vi "TH_Ini_ReadParameters.vi"() -> (19 "error out":errorcluster)   [LabVIEW 2020]
uses:
  TH_StartParameters.vi
  <vilib>/Utility/config.llb/Read Key (String).vi
  TH_Ini_Parameters.vi
  <vilib>/Utility/config.llb/Read Key (Boolean).vi
  <vilib>/Utility/config.llb/Read Key (I32).vi
  <vilib>/Utility/config.llb/NI_LVConfig.lvlib
panel:
  out "Inifile Path":path
  out "Vi Path":path
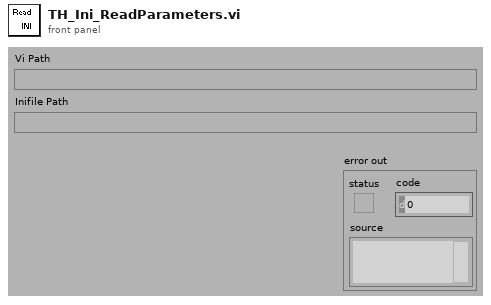
[diagram p1: front panel]
types:
  T1 = typedef "NI_LVConfig.lvlib/Config Data RefNum.ctl" = refnum<k1>
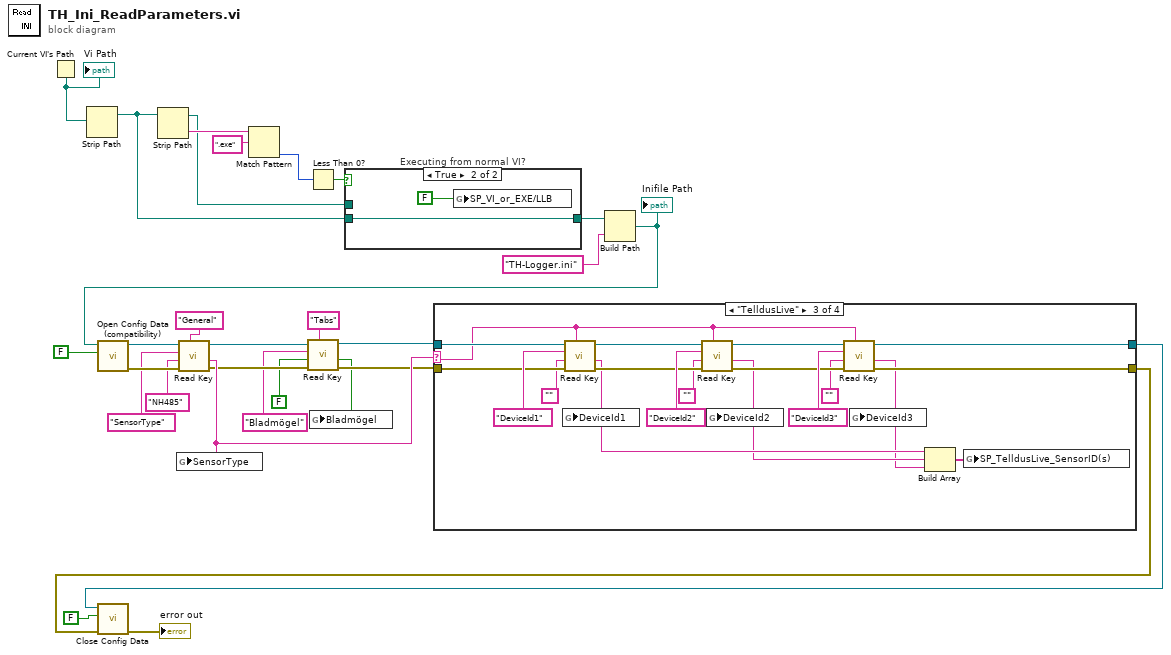
[diagram p0: block diagram]
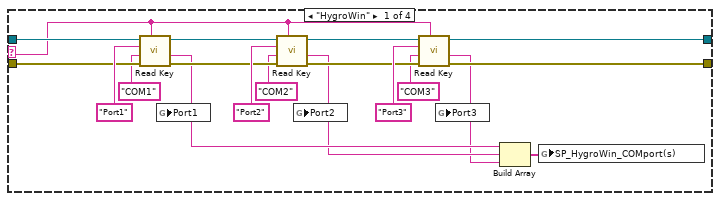
[diagram p2: hidden frame]
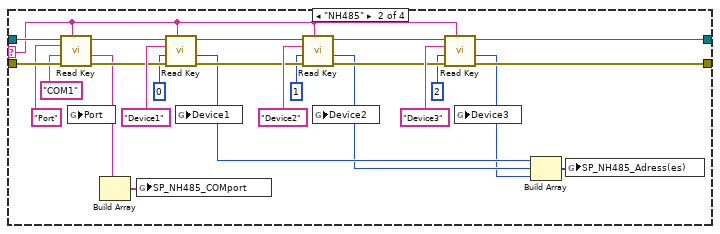
[diagram p3: hidden frame]
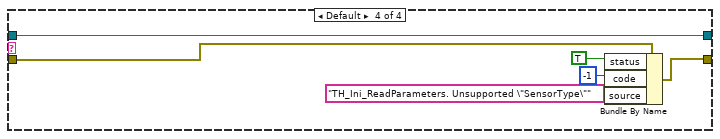
[diagram p4: hidden frame]
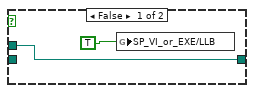
[diagram p5: hidden frame]
diagram:
  n1 = Current VI's Path() -> (path=w27:path)
  "Vi Path" <- w27
  n2 = Strip Path(path=w27) -> (stripped path=w24:path)  [unwired: 1 out]
  n3 = Strip Path(path=w24) -> (stripped path=w23:path, name=w29:string)
  n4 = Match Pattern(string=w29, regular expression=".exe") -> (offset past match=w25:i32)  [unwired: 1 in, 3 out]
  n5 = Less Than 0?(x=w25) -> (x < 0?=w26:bool)
  n6 = case "Executing from normal VI?" shown="True" w26 {
    tunnel: w24 -> [_ w33]
    tunnel: w23 -> [w31 _]
    tunnel: [w31 w33] -> w22
    frame False {
      n7 = global write "TH_StartParameters.vi" "SP_VI_or_EXE/LLB"(TRUE) -> ()
    }
    frame True {
      n8 = global write "TH_StartParameters.vi" "SP_VI_or_EXE/LLB"(FALSE) -> ()
    }
  }
  n9 = Build Path(base path=w22, name or relative path="TH-Logger.ini") -> (appended path=w18:path)
  "Inifile Path" <- w18
  n10 = call <vilib>:"Open Config Data (compatibility).vi"("create file if necessary (T)"=FALSE ("create file if necessary? (T)"), "configuration file path"=w18) -> ("error out"=w17:errorcluster, "refnum"=w16:T1)  [unwired: 7 in, 1 out]
  n11 = call-poly <vilib>:"Read Key.vi"("section"="General", "error in (no error)"=w17, "default value"="NH485", "key"="SensorType", "refnum"=w16) -> ("error out"=w7:errorcluster, "value"=w14:string, "refnum out"=w10:T1)  [unwired: 3 in, 1 out]
  n12 = global write "TH_Ini_Parameters.vi" "SensorType"(w14) -> ()
  n13 = call-poly <vilib>:"Read Key.vi"("section"="Tabs", "error in (no error)"=w7, "default value"=FALSE, "key"="Bladmögel", "refnum"=w10) -> ("error out"=w8:errorcluster, "value"=w4:bool, "refnum out"=w9:T1)  [unwired: 3 in, 1 out]
  n14 = global write "TH_Ini_Parameters.vi" "Bladmögel"(w4) -> ()
  n15 = case shown="\"TelldusLive\"" w14 {
    selector: w14 -> [w43 w63 w87 _]
    tunnel: w9 -> [w45 w77 w89 w102]
    tunnel: w8 -> [w44 w76 w88 w100]
    tunnel: [w42 w65 w86 w102] -> w12
    tunnel: [w41 w64 w85 w101] -> w13
    frame "HygroWin" {
      n16 = call-poly <vilib>:"Read Key.vi"("section"=w43, "error in (no error)"=w44, "default value"="COM1", "key"="Port1", "refnum"=w45) -> ("error out"=w49:errorcluster, "value"=w40:string, "refnum out"=w50:T1)  [unwired: 3 in, 1 out]
      n17 = global write "TH_Ini_Parameters.vi" "Port1"(w40) -> ()
      n18 = call-poly <vilib>:"Read Key.vi"("section"=w43, "error in (no error)"=w49, "default value"="COM2", "key"="Port2", "refnum"=w50) -> ("error out"=w46:errorcluster, "value"=w39:string, "refnum out"=w47:T1)  [unwired: 3 in, 1 out]
      n19 = global write "TH_Ini_Parameters.vi" "Port2"(w39) -> ()
      n20 = call-poly <vilib>:"Read Key.vi"("section"=w43, "error in (no error)"=w46, "default value"="COM3", "key"="Port3", "refnum"=w47) -> ("error out"=w41:errorcluster, "value"=w38:string, "refnum out"=w42:T1)  [unwired: 3 in, 1 out]
      n21 = global write "TH_Ini_Parameters.vi" "Port3"(w38) -> ()
      n22 = Build Array(w40, w39, w38) -> (w37:string[])
      n23 = global write "TH_StartParameters.vi" "SP_HygroWin_COMport(s)"(w37) -> ()
    }
    frame "NH485" {
      n24 = call-poly <vilib>:"Read Key.vi"("section"=w63, "error in (no error)"=w76, "default value"="COM1", "key"="Port", "refnum"=w77) -> ("error out"=w72:errorcluster, "value"=w62:string, "refnum out"=w73:T1)  [unwired: 3 in, 1 out]
      n25 = global write "TH_Ini_Parameters.vi" "Port"(w62) -> ()
      n26 = Build Array(w62, w62, w62) -> (w61:string[])
      n27 = global write "TH_StartParameters.vi" "SP_NH485_COMport"(w61) -> ()
      n28 = call-poly <vilib>:"Read Key.vi"("section"=w63, "error in (no error)"=w72, "default value"=0, "key"="Device1", "refnum"=w73) -> ("error out"=w69:errorcluster, "value"=w60:i32, "refnum out"=w70:T1)  [unwired: 3 in, 1 out]
      n29 = global write "TH_Ini_Parameters.vi" "Device1"(w60) -> ()
      n30 = call-poly <vilib>:"Read Key.vi"("section"=w63, "error in (no error)"=w69, "default value"=1, "key"="Device2", "refnum"=w70) -> ("error out"=w66:errorcluster, "value"=w59:i32, "refnum out"=w67:T1)  [unwired: 3 in, 1 out]
      n31 = global write "TH_Ini_Parameters.vi" "Device2"(w59) -> ()
      n32 = call-poly <vilib>:"Read Key.vi"("section"=w63, "error in (no error)"=w66, "default value"=2, "key"="Device3", "refnum"=w67) -> ("error out"=w64:errorcluster, "value"=w58:i32, "refnum out"=w65:T1)  [unwired: 3 in, 1 out]
      n33 = global write "TH_Ini_Parameters.vi" "Device3"(w58) -> ()
      n34 = Build Array(w60, w59, w58) -> (w57:i32[])
      n35 = global write "TH_StartParameters.vi" "SP_NH485_Adress(es)"(w57) -> ()
    }
    frame "TelldusLive" {
      n36 = call-poly <vilib>:"Read Key.vi"("section"=w87, "error in (no error)"=w88, "default value"="", "key"="DeviceId1", "refnum"=w89) -> ("error out"=w93:errorcluster, "value"=w84:string, "refnum out"=w94:T1)  [unwired: 3 in, 1 out]
      n37 = global write "TH_Ini_Parameters.vi" "DeviceId1"(w84) -> ()
      n38 = call-poly <vilib>:"Read Key.vi"("section"=w87, "error in (no error)"=w93, "default value"="", "key"="DeviceId2", "refnum"=w94) -> ("error out"=w90:errorcluster, "value"=w83:string, "refnum out"=w91:T1)  [unwired: 3 in, 1 out]
      n39 = global write "TH_Ini_Parameters.vi" "DeviceId2"(w83) -> ()
      n40 = call-poly <vilib>:"Read Key.vi"("section"=w87, "error in (no error)"=w90, "default value"="", "key"="DeviceId3", "refnum"=w91) -> ("error out"=w85:errorcluster, "value"=w82:string, "refnum out"=w86:T1)  [unwired: 3 in, 1 out]
      n41 = global write "TH_Ini_Parameters.vi" "DeviceId3"(w82) -> ()
      n42 = Build Array(w84, w83, w82) -> (w81:string[])
      n43 = global write "TH_StartParameters.vi" "SP_TelldusLive_SensorID(s)"(w81) -> ()
    }
    frame Default {
      n44 = Bundle By Name(cluster=w100, "status"=TRUE, "code"=-1, "source"="TH_Ini_ReadParameters. Unsupported \"SensorType\"") -> (w101:errorcluster)
    }
  }
  n45 = call <vilib>:"Close Config Data.vi"("error in (no error)"=w13, "write file if changed (T)"=FALSE ("write configuration file? (T)"), "refnum"=w12) -> ("error out"=→"error out":errorcluster)  [unwired: 7 in, 1 out]
